vi "get sys config device information.vi"(8 "error in":errorcluster, 11 "syscfg device in":refnum<class "SysCfg Device.lvclass">) -> (0 "error out":errorcluster, 2 "device information":T1 {"product ID" format="%.0x"}, 3 "syscfg device out":refnum<class "SysCfg Device.lvclass">)   [LabVIEW 2014, in "SMI.lvlib" / "SysCfg Device.lvclass"]
uses:
  SysCfg Device.lvclass
  sys config device information.ctl
  Device/read serial number.vi
  Device/read product ID.vi
  Device/read product name.vi
  Device/read vendor name.vi
  read system session.vi
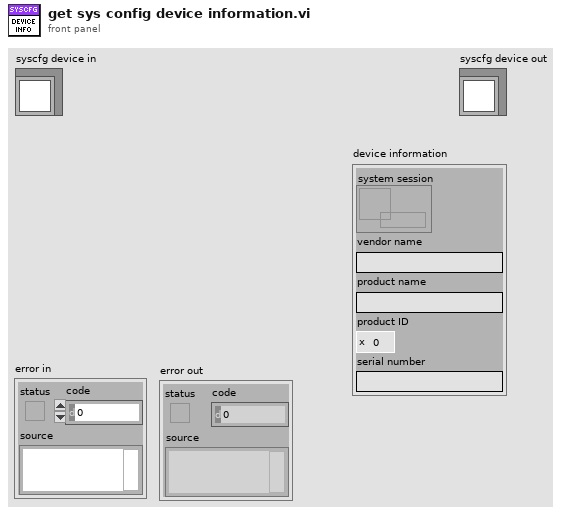
[diagram p1: front panel]
types:
  T1 = typedef "SMI.lvlib/SysCfg Device.lvclass/sys config device information.ctl" = cluster{"system session":refnum<data-value>, "vendor name":string, "product name":string, "product ID":u32, "serial number":string}
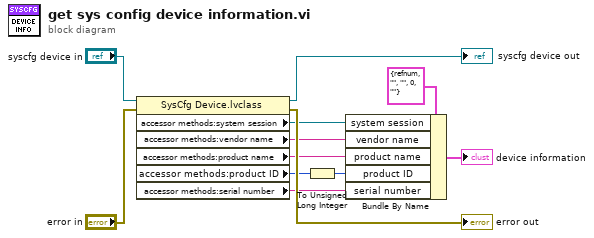
[diagram p0: block diagram]
diagram:
  n1 = property class="SysCfg Device.lvclass"(reference="syscfg device in", error in="error in") -> (reference out=→"syscfg device out":refnum<class "SysCfg Device.lvclass">, error out=→"error out":errorcluster, "accessor methods:system session"=w6:refnum<data-value>, "accessor methods:vendor name"=w5:string, "accessor methods:product name"=w4:string, "accessor methods:product ID"=w1:u16, "accessor methods:serial number"=w3:string)
  n2 = To Unsigned Long Integer(number=w1) -> (unsigned 32bit integer=w2:u32)
  n3 = Bundle By Name(cluster=T1 {"system session"=refnum, "vendor name"="", "product name"="", "product ID"=0, "serial number"=""} ("Device Information"), "system session"=w6, "vendor name"=w5, "product name"=w4, "product ID"=w2, "serial number"=w3) -> (→"device information":T1)
